vi "publish.vi"(6 "retain":bool, 8 "Error In":errorcluster, 9 "payload (something)":string="something", 10 "qos (1)":i32=1, 11 "topic (test/device1)":string="test/device1") -> (0 "Error Out":errorcluster)   [LabVIEW 2016, in "mqtt.lvlib"]
uses:
  mqtt.lvlib
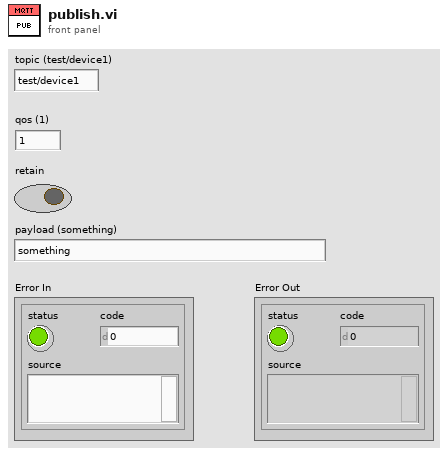
[diagram p1: front panel]
types:
  T1 = cluster{"command":string, "topic":string, "payload":string, "qos":i32, "retain":bool}
  T2 = enum16{"big-endian, network order", "native, host order", "little-endian"}
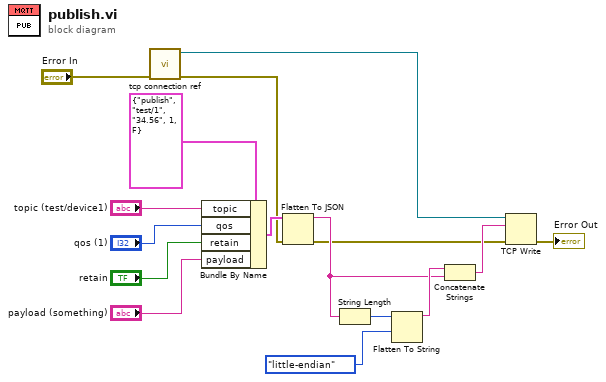
[diagram p0: block diagram]
diagram:
  n1 = call "tcp connection ref.vi"("Error In"="Error In") -> ("Error Out"=w7:errorcluster, "tcpRef"=w5:refnum<k5>)  [unwired: 9 in]
  n2 = Bundle By Name(cluster=T1 {"command"="publish", "topic"="test/1", "payload"="34.56", "qos"=1, "retain"=FALSE} ("publish"), "topic"="topic (test/device1)", "qos"="qos (1)", "retain"="retain", "payload"="payload (something)") -> (w10:T1)
  n3 = Flatten To JSON(anything=w10, error in (no error)=w7) -> (JSON string=w9:string, 11:w6:errorcluster)  [unwired: 1 in]
  n4 = String Length(string=w9) -> (length=w13:i32)
  n5 = Flatten To String(anything=w13, byte order (0:big-endian, network order)=T2."little-endian") -> (data string=w12:string)  [unwired: 2 in, 2 out]
  n6 = Concatenate Strings(w12, w9) -> (w11:string)
  n7 = TCP Write(connection ID=w5, data in=w11, error in (no error)=w6) -> (error out=→"Error Out":errorcluster)  [unwired: 1 in, 2 out]
